vi "Get Data (Filtered).vi"(8 "error in (no error)":errorcluster, 10 "Filter Value (T)":bool=TRUE, 11 "MCListbox with Checkboxes in":refnum<class "MCListbox with Checkboxes.lvclass">) -> (0 "error out":errorcluster, 2 "Cell Data":string[][](array[string]), 3 "MCListbox with Checkboxes out":refnum<class "MCListbox with Checkboxes.lvclass">)   [LabVIEW 2016, in "MCListbox with Checkboxes.lvclass"]
uses:
  MCListbox with Checkboxes.lvclass
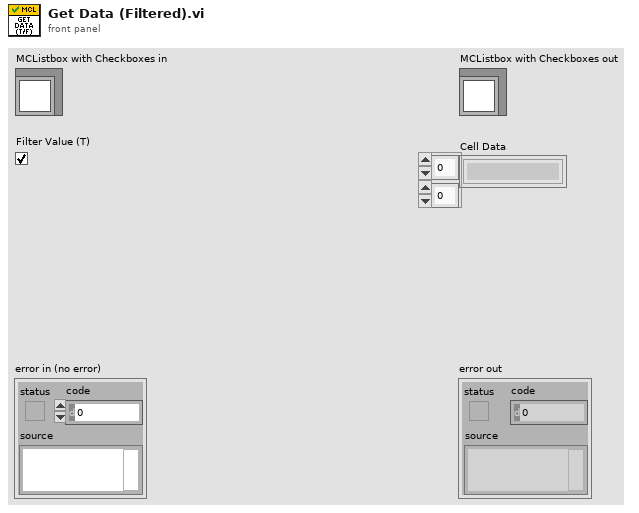
[diagram p1: front panel]
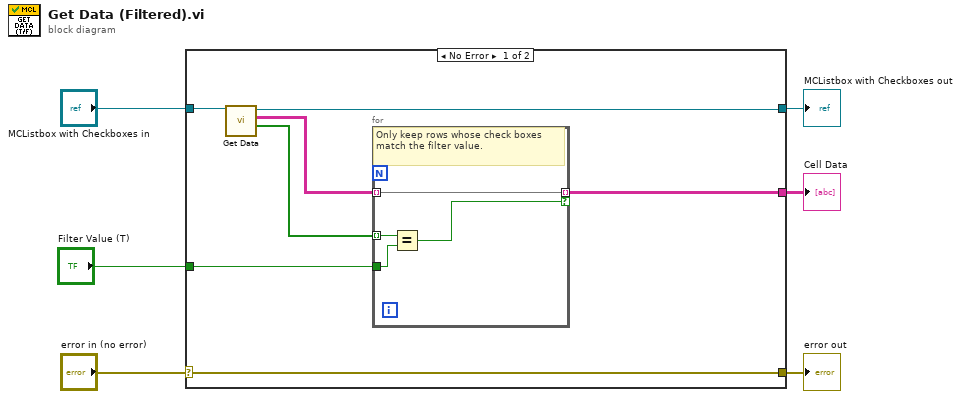
[diagram p0: block diagram]
diagram:
  n1 = case shown="No Error" "error in (no error)" {
    selector: "error in (no error)" -> [w13 w19]
    tunnel: [w13 w19] -> w5
    tunnel: [w11 w18] -> w3
    tunnel: "MCListbox with Checkboxes in" -> [w12 w18]
    tunnel: "Filter Value (T)" -> [w8 _]
    tunnel: [w7 _] -> w1
    frame No Error {
      n2 = call "Get Data.vi"("MCListbox with Checkboxes in"=w12) -> ("Check Data"=w9:bool[], "Cell Data"=w10:string[][], "MCListbox with Checkboxes out"=w11:refnum<class "MCListbox with Checkboxes.lvclass">)  [unwired: 7 in, 1 out]
      n3 = for {
        tunnel: w10 -> [w15] mode=indexing
        tunnel: w9 -> [w17] mode=indexing
        tunnel: w8 -> [w16]
        tunnel: [w15] -> w7 mode=indexing if=w14
        # "Only keep rows whose check boxes match the filter value."
        n4 = Equal?(x=w17, y=w16) -> (x = y?=w14:bool)
      }
    }
    frame Error {
    }
  }
  "error out" <- w5
  "MCListbox with Checkboxes out" <- w3
  "Cell Data" <- w1
